vi "tinyraytracer.vi"() -> ()   [LabVIEW 2015]
uses:
  Sphere.ctl
  Material.ctl
  Light.ctl
  <vilib>/Analysis/_algsub.llb/Real Vector Norm.vi
  <vilib>/picture/picture.llb/Draw True-Color Pixmap.vi
  <vilib>/Analysis/NI_AALPro.lvlib
panel:
  out "picture":picture
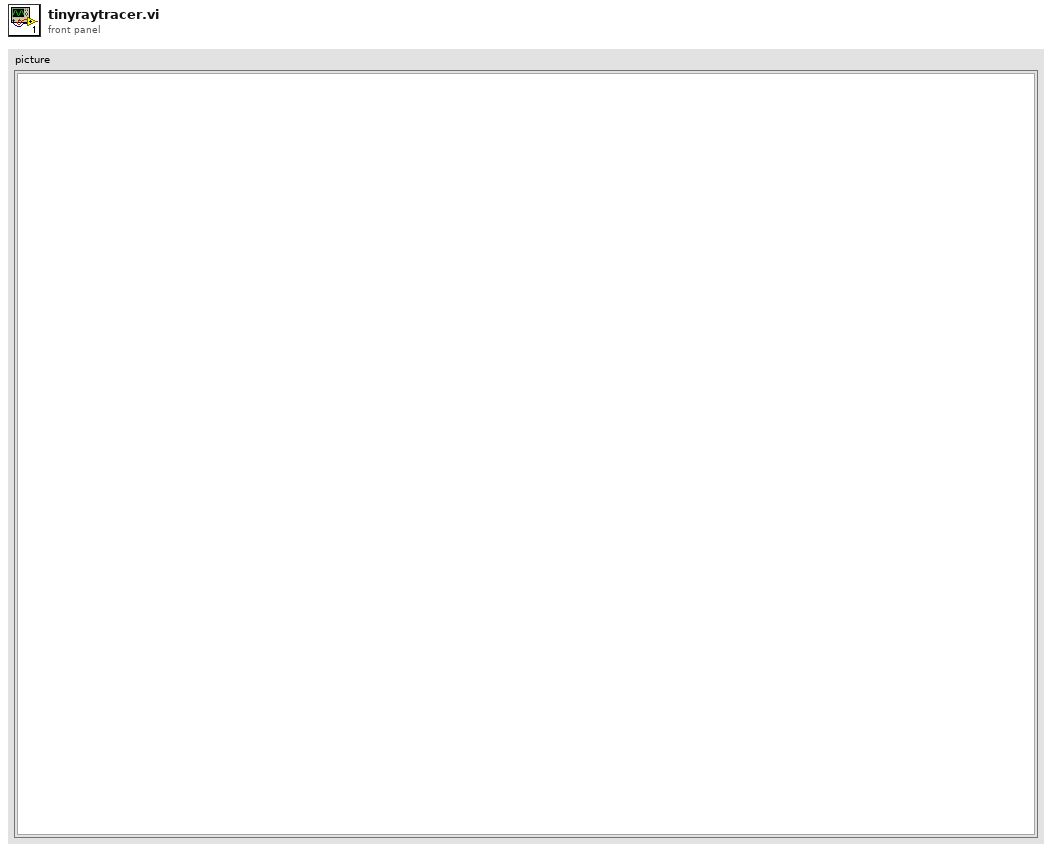
[diagram p1: front panel]
types:
  T1 = typedef "Light.ctl" = cluster{"Position":dbl[], "Intencity":dbl}
  T2 = typedef "Sphere.ctl" = cluster{"Center":dbl[], "Radius":dbl, "Material":T3}
  T3 = typedef "Material.ctl" = cluster{"Albedo":dbl[], "DiffuseColor":u32, "SpecularExp":dbl, "RefractInd":dbl}
  T4 = typedef "imagedata.ctl" = cluster{"image type":i32, "image depth":i32, "image":u8[], "mask":u8[], "colors":u32[], "Rectangle":cluster{"left":i16, "top":i16, "right":i16, "bottom":i16}}
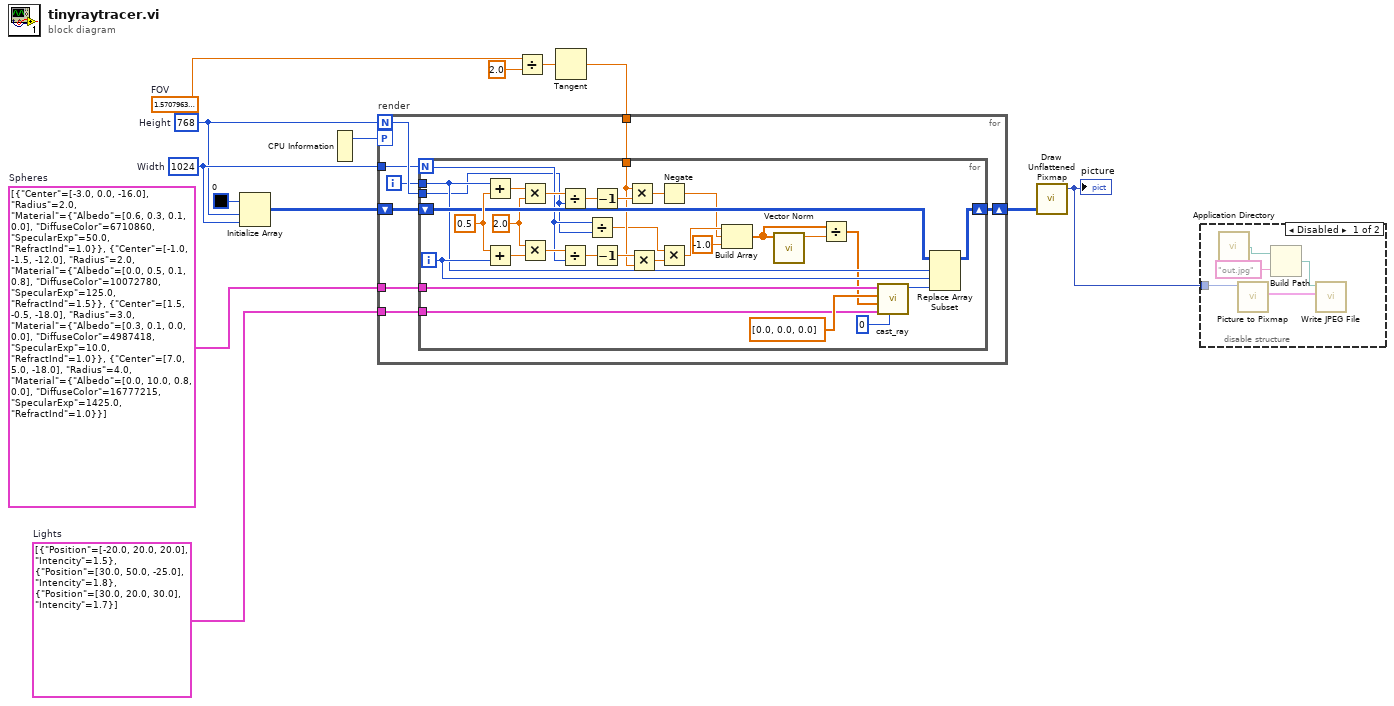
[diagram p0: block diagram]
diagram:
  w2 = T1[] [{"Position"=[-20.0, 20.0, 20.0], "Intencity"=1.5}, {"Position"=[30.0, 50.0, -25.0], "Intencity"=1.8}, {"Position"=[30.0, 20.0, 30.0], "Intencity"=1.7}]  # Lights
  w3 = T2[] [{"Center"=[-3.0, 0.0, -16.0], "Radius"=2.0, "Material"={"Albedo"=[0.6, 0.3, 0.1, 0.0], "DiffuseColor"=6710860, "SpecularExp"=50.0, "RefractInd"=1.0}}, {"Center"=[-1.0, -1.5, -12.0], "Radius"=2.0, "Material"={"Albedo"=[0.0, 0.5, 0.1, 0.8], "DiffuseColor"=10072780, "SpecularExp"=125.0, "RefractInd"=1.5}}, {"Center"=[1.5, -0.5, -18.0], "Radius"=3.0, "Material"={"Albedo"=[0.3, 0.1, 0.0, 0.0], "DiffuseColor"=4987418, "SpecularExp"=10.0, "RefractInd"=1.0}}, {"Center"=[7.0, 5.0, -18.0], "Radius"=4.0, "Material"={"Albedo"=[0.0, 10.0, 0.8, 0.0], "DiffuseColor"=16777215, "SpecularExp"=1425.0, "RefractInd"=1.0}}]  # Spheres
  w7 = 1.5707963267948966  # FOV
  w9 = 768  # Height
  w10 = 1024  # Width
  n1 = Initialize Array(u32 0 ("Color"), w9, w10) -> (w12:u32[][])
  n2 = CPU Information() -> (4:w1:i32)  [unwired: 3 out]
  n3 = Divide(x=w7, y=2.0) -> (x/y=w5:dbl)
  n4 = Tangent(1:w5) -> (0:w4:dbl)
  n5 = for "render" {
    N: w9 -> [w21]
    tunnel: w10 -> [w20]
    shift-right: [w18] -> w11
    shift-left: w12 -> [w19]
    tunnel: w3 -> [w15]
    tunnel: w4 -> [w16]
    tunnel: w2 -> [w14]
    workers-P: w1 -> [_]
    i -> [w17]
    n6 = for {
      N: w20 -> [w37]
      shift-right: [w52] -> w18
      shift-left: w19 -> [w50]
      tunnel: w21 -> [w36]
      tunnel: w17 -> [w48]
      tunnel: w15 -> [w28]
      tunnel: w16 -> [w38]
      tunnel: w14 -> [w23]
      i -> [w49]
      w45 = 2.0
      w51 = 0.5
      n7 = Add(x=w48, y=w51) -> (x+y=w46:dbl)
      n8 = Add(x=w51, y=w49) -> (x+y=w47:dbl)
      n9 = Multiply(x=w46, y=w45) -> (x*y=w44:dbl)
      n10 = Multiply(x=w45, y=w47) -> (x*y=w43:dbl)
      n11 = Divide(x=w44, y=w36) -> (x/y=w42:dbl)
      n12 = Divide(x=w43, y=w37) -> (x/y=w41:dbl)
      n13 = Divide(x=w37, y=w36) -> (x/y=w34:dbl)
      n14 = Decrement(x=w42) -> (x-1=w40:dbl)
      n15 = Decrement(x=w41) -> (x-1=w39:dbl)
      n16 = Multiply(x=w38, y=w40) -> (x*y=w33:dbl)
      n17 = Multiply(x=w39, y=w38) -> (x*y=w35:dbl)
      n18 = Negate(x=w33) -> (-x=w24:dbl)
      n19 = Multiply(x=w34, y=w35) -> (x*y=w32:dbl)
      n20 = Build Array(w32, w24, -1.0 ("element")) -> (w29:dbl[])
      n21 = call-poly <vilib>:"Vector Norm.vi"("Input Vector"=w29) -> ("norm"=w30:dbl)  [unwired: 9 in, 1 out]
      n22 = Divide(x=w29, y=w30) -> (x/y=w26:dbl[])
      n23 = call "cast_ray.vi"("Depth"=0, "Lights"=w23, "Direction"=w26, "Origin"=dbl[] [0.0, 0.0, 0.0], "Spheres"=w28) -> ("Color"=w25:u32)  [unwired: 6 in]
      n24 = Replace Array Subset(array=w50, new element=w25, index (row)=w48, index (col)=w49) -> (w52:u32[][])
    }
  }
  n25 = call-poly <vilib>:"Draw Unflattened Pixmap.vi"("data (RGB format)"=w11) -> ("new picture"=w8:picture)  [unwired: 8 in]
  "picture" <- w8
  n26 = disable-structure shown="Disabled" {
    disable-tunnel: w8 -> [w57 _]
    frame Disabled {
      n27 = call <vilib>:"Application Directory.vi"() -> ("Application Directory"=w54:path)
      n28 = call <vilib>:"Picture to Pixmap.vi"("picture"=w57) -> ("image data"=w56:T4)  [unwired: 9 in, 1 out]
      n29 = Build Path(base path=w54, name or relative path="out.jpg") -> (appended path=w53:path)
      n30 = call <vilib>:"Write JPEG File.vi"("image data"=w56, "path to JPEG file"=w53) -> ()  [unwired: 8 in, 2 out]
    }
    frame Enabled {
    }
  }
